vi "overlay enum on cell.vi"(4 "cell position":T1, 7 "Overlay?":bool, 8 "error in":errorcluster, 9 "Table Reference":refnum<vi>, 10 "current value":T2, 11 "Enum in":refnum<vi>) -> (0 "error out":errorcluster)   [LabVIEW 2013]
uses:
  <vilib>/NI/Tag Bus/tag/Data Type.ctl
  <vilib>/Utility/miscctls.llb/LVRowAndColumnTypeDef.ctl
  <vilib>/Utility/miscctls.llb/LVPositionTypeDef.ctl
  <vilib>/NI/Tag Bus Data Framework/Configuration Editor/Classes/EngineTags/EngineTags.lvclass
  <vilib>/NI/Tag Bus/tag/tag descriptor.lvclass
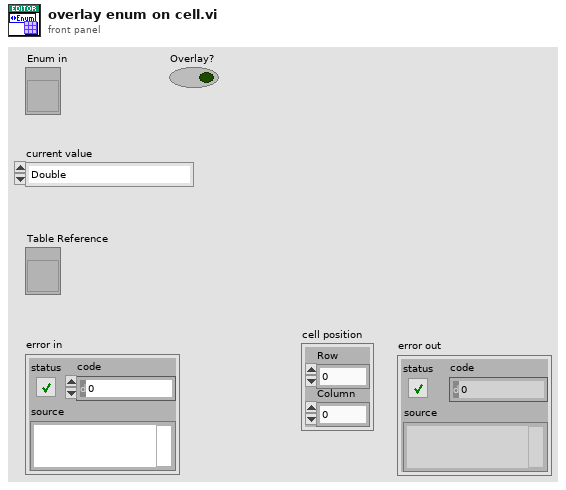
[diagram p1: front panel]
types:
  T1 = typedef "LVRowAndColumnTypeDef.ctl" = cluster{"Row":i32, "Column":i32}
  T2 = typedef "tag bus.lvlib/tag descriptor.lvclass/Data Type.ctl" = enum16{"Double", "Single", "I64", "I32", "I16", "I8", "U64", "U32", "U16", "U8", "Boolean", "String", "Array of Double", "Array of Single", "Array of I64", "Array of I32", "Array of I16", "Array of I8", "Array of U64", "Array of U32", "Array of U16", "Array of U8", "Array of Boolean", "Array of String"}
  T3 = typedef "LVPositionTypeDef.ctl" = cluster{"Left":i32, "Top":i32}
  T4 = typedef "LVBoundsTypeDef.ctl" = cluster{"Width":u32, "Height":u32}
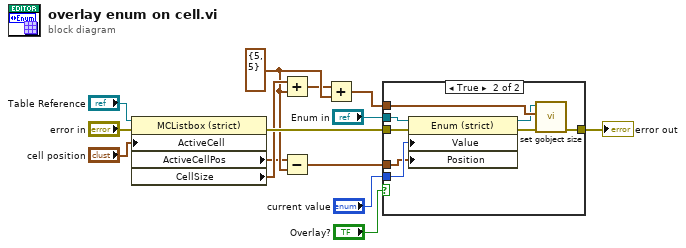
[diagram p0: block diagram]
diagram:
  w6 = T3 {"Left"=5, "Top"=5} ("Active Cell:Position")
  n1 = property class="MCListbox (strict)"(reference="Table Reference", error in="error in", "ActiveCell"="cell position") -> (error out=w12:errorcluster, "ActiveCellPos"=w5:T3, "CellSize"=w7:T4)  [unwired: 1 out]
  n2 = Add(x=w7, y=w6) -> (x+y=w3:T4)
  n3 = Subtract(x=w5, y=w6) -> (x-y=w13:T3)
  n4 = Add(x=w3, y=w6) -> (x+y=w4:T4)
  n5 = case shown="True" "Overlay?" {
    tunnel: w12 -> [w15 w19]
    tunnel: [w15 w23] -> w1
    tunnel: w4 -> [_ w22]
    tunnel: "current value" -> [_ w20]
    tunnel: w13 -> [_ w17]
    tunnel: "Enum in" -> [_ w16]
    frame False {
    }
    frame True {
      n6 = property on="Property Node" class="Enum (strict)"(reference=w16, error in=w19, "Value"=w20, "Position"=w17) -> (reference out=w21:refnum<vi>, error out=w18:errorcluster)
      n7 = call <vilib>:"set gobject size.vi"("error in"=w18, "size"=w22, "object refnum"=w21) -> ("error out"=w23:errorcluster)  [unwired: 8 in]
    }
  }
  "error out" <- w1
